vi "NameData_Select Format String.vi"(6 "Data Type":T2, 8 "Error":errorcluster, 9 "Format Cluster":T3, 11 "String Format Select":T1) -> (0 "Error Out":errorcluster, 3 "Format String Out":string)   [LabVIEW 2015]
uses:
  TypeDefs_Utility/Cluster_NameData_String Format Data.ctl
  <vilib>/Utility/VariantDataType/Type.ctl
  TypeDefs_Utility/ENUM_NameData_String Format Select.ctl
  <vilib>/Utility/VariantDataType/VariantType.lvlib
panel:
  # "%.2f %g %e %p"
  # "%d %h %o %b"
  # "'%s'"
  # "%x %X"
  # "True,False -1,0 Yes,No"
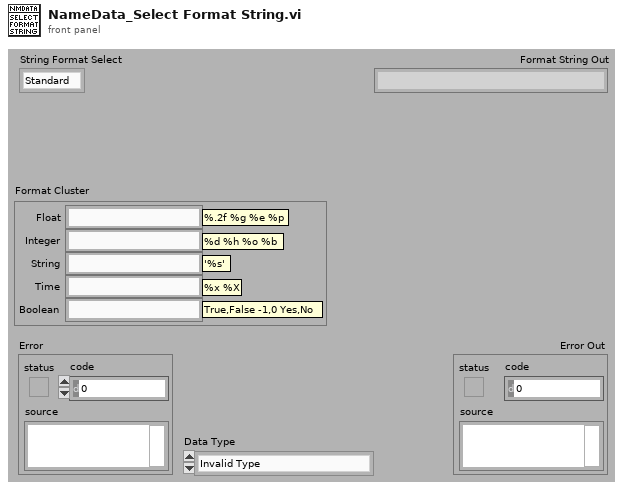
[diagram p1: front panel]
types:
  T1 = typedef "ENUM_NameData_String Format Select.ctl" = enum16{"Standard", "Access DB", "Custom"}
  T2 = typedef "VariantType.lvlib/Type.ctl" = enum8{"Invalid Type", "Void", "I8", "I16", "I32", "I64", "U8", "U16", "U32", "U64", "Single Float", "Double Float", "Extended Float", "Single Complex", "Double Complex", "Extended Complex", "Enum U8", "Enum U16", "Enum U32", "Enum U64", "Single Float With Unit", "Double Float With Unit", "Extended Float With Unit", "Single Complex with Unit", "Double Complex with Unit", "Extended Complex with Unit", "Boolean", "String", "Path", "Picture", "Tag", "Array", "Cluster", "Variant", "LV Variant", "Waveform", "Timestamp", "Digital Waveform", "Digital Data", "ExpressData", "Refnum", "External Data", "VI", "Poly VI", "LabVIEW Class Instance", "Fixed Point"}
  T3 = typedef "Cluster_NameData_String Format Data.ctl" = cluster{"Float":string, "Integer":string, "String":string, "Time":string, "Boolean":string}
  T4 = cluster{"[0]":string, "[1]":string, "[2]":string, "[3]":string, "[4]":string}
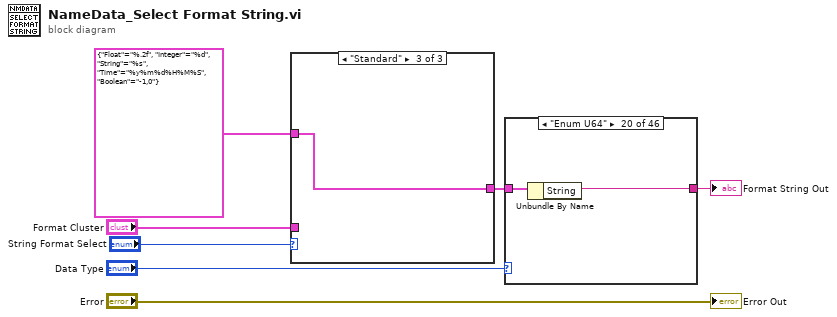
[diagram p0: block diagram]
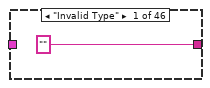
[diagram p2: hidden frame]
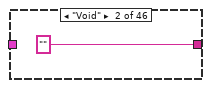
[diagram p3: hidden frame]
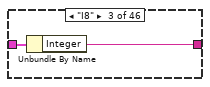
[diagram p4: hidden frame]
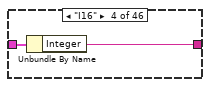
[diagram p5: hidden frame]
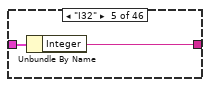
[diagram p6: hidden frame]
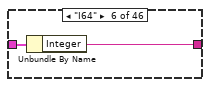
[diagram p7: hidden frame]
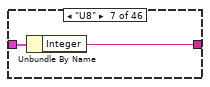
[diagram p8: hidden frame]
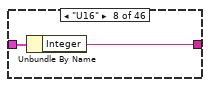
[diagram p9: hidden frame]
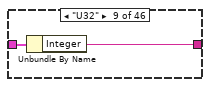
[diagram p10: hidden frame]
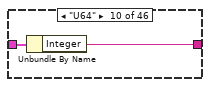
[diagram p11: hidden frame]
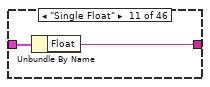
[diagram p12: hidden frame]
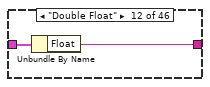
[diagram p13: hidden frame]
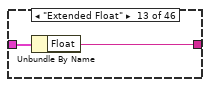
[diagram p14: hidden frame]
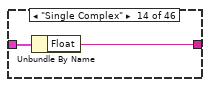
[diagram p15: hidden frame]
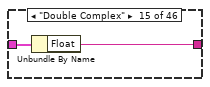
[diagram p16: hidden frame]
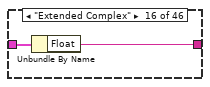
[diagram p17: hidden frame]
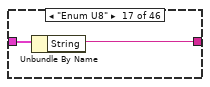
[diagram p18: hidden frame]
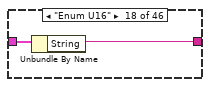
[diagram p19: hidden frame]
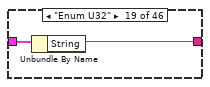
[diagram p20: hidden frame]
diagram:
  n1 = case shown="\"Standard\"" "String Format Select" {
    tunnel: "Format Cluster" -> [_ w13 _]
    tunnel: T3 {"Float"="%.2f", "Integer"="%d", "String"="%s", "Time"="%y%m%d%H%M%S", "Boolean"="-1,0"} ("Format Cluster") -> [_ w14 w19]
    tunnel: [T3 {"Float"="%.2f", "Integer"="%d", "String"="'%s'", "Time"="'%x %X'", "Boolean"="-1,0"} ("Format Cluster") w9 w19] -> w2
    frame "Access DB" {
    }
    frame "Custom" {
      n2 = Cluster To Array(cluster=w14) -> (array=w11:string[])
      n3 = Cluster To Array(cluster=w13) -> (array=w12:string[])
      n4 = for {
        tunnel: w12 -> [w16] mode=indexing
        tunnel: w11 -> [w17] mode=indexing
        tunnel: [w15] -> w10 mode=indexing
        n5 = Empty String/Path?(string/path=w16) -> (empty?=w18:bool)
        n6 = Select(t=w17, s=w18, f=w16) -> (s? t:f=w15:string)
      }
      n7 = Array To Cluster(array=w10) -> (cluster=w9:T4)
    }
    frame "Standard" {
    }
  }
  n8 = case shown="\"Enum U64\"" "Data Type" {
    tunnel: w2 -> [_ _ w23 w25 w27 w29 w31 w33 w35 w37 w39 w41 w43 w45 w47 w49 w51 w53 w55 w57 w59 w61 w63 w65 w67 w69 w71 w73 w75 _ w78 _ _ _ _ w84 w86 w88 w90 _ w93 _ _ _ _ w99]
    tunnel: ["" "" w22 w24 w26 w28 w30 w32 w34 w36 w38 w40 w42 w44 w46 w48 w50 w52 w54 w56 w58 w60 w62 w64 w66 w68 w70 w72 w74 "" ("String") w77 "" ("String") "" ("String") "" ("String") "" ("String") w83 w85 w87 w89 "" ("Boolean") w92 "" ("Integer") "" ("Integer") "" ("Integer") "" ("Integer") w98] -> w1
    frame "Invalid Type" {
    }
    frame "Void" {
    }
    frame "I8" {
      n9 = Unbundle By Name(w23) -> ("Integer"=w22:string)
    }
    frame "I16" {
      n10 = Unbundle By Name(w25) -> ("Integer"=w24:string)
    }
    frame "I32" {
      n11 = Unbundle By Name(w27) -> ("Integer"=w26:string)
    }
    frame "I64" {
      n12 = Unbundle By Name(w29) -> ("Integer"=w28:string)
    }
    frame "U8" {
      n13 = Unbundle By Name(w31) -> ("Integer"=w30:string)
    }
    frame "U16" {
      n14 = Unbundle By Name(w33) -> ("Integer"=w32:string)
    }
    frame "U32" {
      n15 = Unbundle By Name(w35) -> ("Integer"=w34:string)
    }
    frame "U64" {
      n16 = Unbundle By Name(w37) -> ("Integer"=w36:string)
    }
    frame "Single Float" {
      n17 = Unbundle By Name(w39) -> ("Float"=w38:string)
    }
    frame "Double Float" {
      n18 = Unbundle By Name(w41) -> ("Float"=w40:string)
    }
    frame "Extended Float" {
      n19 = Unbundle By Name(w43) -> ("Float"=w42:string)
    }
    frame "Single Complex" {
      n20 = Unbundle By Name(w45) -> ("Float"=w44:string)
    }
    frame "Double Complex" {
      n21 = Unbundle By Name(w47) -> ("Float"=w46:string)
    }
    frame "Extended Complex" {
      n22 = Unbundle By Name(w49) -> ("Float"=w48:string)
    }
    frame "Enum U8" {
      n23 = Unbundle By Name(w51) -> ("String"=w50:string)
    }
    frame "Enum U16" {
      n24 = Unbundle By Name(w53) -> ("String"=w52:string)
    }
    frame "Enum U32" {
      n25 = Unbundle By Name(w55) -> ("String"=w54:string)
    }
    frame "Enum U64" {
      n26 = Unbundle By Name(w57) -> ("String"=w56:string)
    }
    frame "Single Float With Unit" {
      n27 = Unbundle By Name(w59) -> ("Float"=w58:string)
    }
    frame "Double Float With Unit" {
      n28 = Unbundle By Name(w61) -> ("Float"=w60:string)
    }
    frame "Extended Float With Unit" {
      n29 = Unbundle By Name(w63) -> ("Float"=w62:string)
    }
    frame "Single Complex with Unit" {
      n30 = Unbundle By Name(w65) -> ("Float"=w64:string)
    }
    frame "Double Complex with Unit" {
      n31 = Unbundle By Name(w67) -> ("Float"=w66:string)
    }
    frame "Extended Complex with Unit" {
      n32 = Unbundle By Name(w69) -> ("Float"=w68:string)
    }
    frame "Boolean" {
      n33 = Unbundle By Name(w71) -> ("Boolean"=w70:string)
    }
    frame "String" {
      n34 = Unbundle By Name(w73) -> ("String"=w72:string)
    }
    frame "Path" {
      n35 = Unbundle By Name(w75) -> ("String"=w74:string)
    }
    frame "Picture" {
    }
    frame "Tag" {
      n36 = Unbundle By Name(w78) -> ("String"=w77:string)
    }
    frame "Array" {
    }
    frame "Cluster" {
    }
    frame "Variant" {
    }
    frame "LV Variant" {
    }
    frame "Waveform" {
      n37 = Unbundle By Name(w84) -> ("Float"=w83:string)
    }
    frame "Timestamp" {
      n38 = Unbundle By Name(w86) -> ("Time"=w85:string)
    }
    frame "Digital Waveform" {
      n39 = Unbundle By Name(w88) -> ("Boolean"=w87:string)
    }
    frame "Digital Data" {
      n40 = Unbundle By Name(w90) -> ("Boolean"=w89:string)
    }
    frame "ExpressData" {
    }
    frame "Refnum" {
      n41 = Unbundle By Name(w93) -> ("Integer"=w92:string)
    }
    frame "External Data" {
    }
    frame "VI" {
    }
    frame "Poly VI" {
    }
    frame "LabVIEW Class Instance" {
    }
    frame "Fixed Point" {
      n42 = Unbundle By Name(w99) -> ("Float"=w98:string)
    }
  }
  "Format String Out" <- w1
  "Error Out" <- "Error"
